vi "ServoControl_myrio_v1.vi"() -> ()   [LabVIEW 2019]
uses:
  <vilib>/Instr/_visa.llb/VISA Configure Serial Port (Instr).vi
panel:
  out "Position Chart":dbl(graph)
  out "resulting string":string
  in  "Numeric":dbl
  in  "stop":bool
  out "read buffer":string
  out "error out 2":errorcluster
  in  "Baud rate 2":dbl=500000.0
  in  "VISA resource name 2":refnum<visa-resource-name>
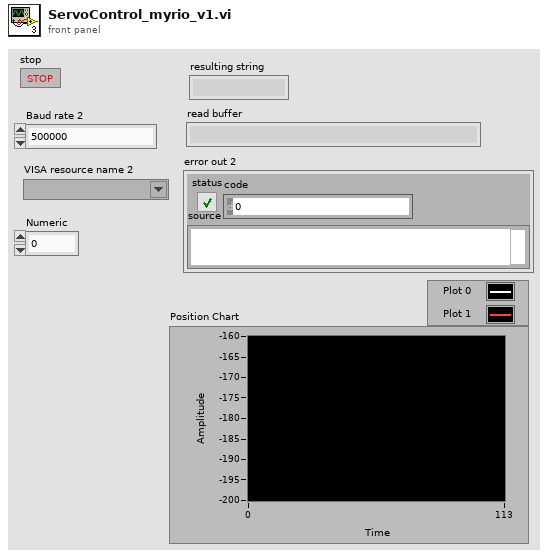
[diagram p1: front panel]
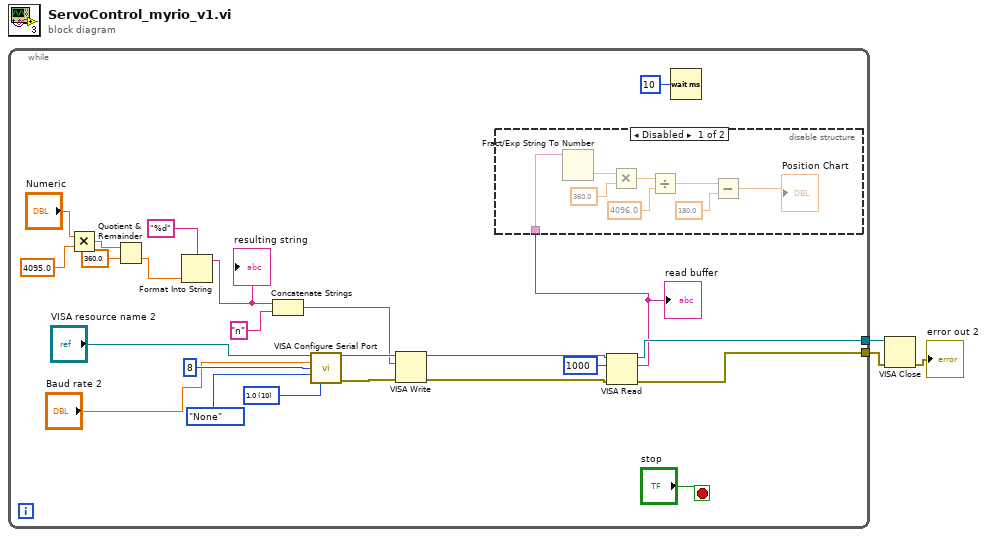
[diagram p0: block diagram]
diagram:
  n1 = while {
    tunnel: [w9] -> w3
    tunnel: [w8] -> w2
    stop <- "stop" stop-if-true
    w23 = u16 10 items=["1.0"=10, "1.5"=15, "2.0"=20] ("stop bits (10: 1 bit)")
    n2 = Multiply(x="Numeric", y=4095.0) -> (x*y=w15:dbl)
    n3 = Quotient & Remainder(x=w15, y=360.0) -> (floor(x/y)=w13:dbl)  [unwired: 1 out]
    n4 = Format Into String(format string="%d", w13) -> (resulting string=w10:string)  [unwired: 2 in, 1 out]
    "resulting string" <- w10
    n5 = Concatenate Strings(w10, "n" ("string")) -> (w19:string)
    n6 = call-poly "VISA Configure Serial Port"("VISA resource name"="VISA resource name 2", "baud rate (9600)"="Baud rate 2", "data bits (8)"=u16 8, "parity (0:none)"=enum16{"None", "Odd", "Even", "Mark", "Space"}."None", "stop bits (10: 1 bit)"=w23) -> ("VISA resource name out"=w22:refnum<visa-resource-name>, "error out"=w21:errorcluster)  [unwired: 9 in]
    n7 = VISA Write(VISA resource name=w22, write buffer=w19, error in (no error)=w21) -> (VISA resource name out=w18:refnum<visa-resource-name>, error out=w17:errorcluster)  [unwired: 1 out]
    n8 = VISA Read(VISA resource name=w18, byte count=u32 1000, error in (no error)=w17) -> (VISA resource name out=w8:refnum<visa-resource-name>, read buffer=w7:string, error out=w9:errorcluster)  [unwired: 1 out]
    "read buffer" <- w7
    n9 = disable-structure shown="Disabled" {
      disable-tunnel: w7 -> [w29 _]
      frame Disabled {
        n10 = Fract/Exp String To Number(string=w29) -> (number=w30:dbl)  [unwired: 3 in, 1 out]
        n11 = Multiply(x=w30, y=360.0 ("x")) -> (x*y=w31:dbl)
        n12 = Divide(x=w31, y=4096.0) -> (x/y=w33:dbl)
        n13 = Subtract(x=w33, y=180.0) -> (x-y=→"Position Chart":dbl)
      }
      frame Enabled {
      }
    }
    n14 = Wait (ms)(milliseconds to wait=u32 10) -> ()  [unwired: 1 out]
  }
  n15 = VISA Close(VISA resource name=w2, error in (no error)=w3) -> (error out=→"error out 2":errorcluster)
